vi "DeviceListCheck.vi"(0 "Device List":string[](array[string])=["9481_1", "9435_1", "9435_2", "9401_1", "9263_1", "9263_2"], 11 "Error In":errorcluster) -> (4 "Devices Present?":bool, 8 "Report Text":string, 15 "Error Out":errorcluster)   [LabVIEW 2023]
uses:
  <vilib>/nisyscfg/Find Hardware.vi
  <vilib>/nisyscfg/Close (System).vi
  <vilib>/nisyscfg/nisyscfg.lvlib
  <resource>/objmgr/nicontrollersysapi.rc
  <resource>/objmgr/pxisysapi.rc
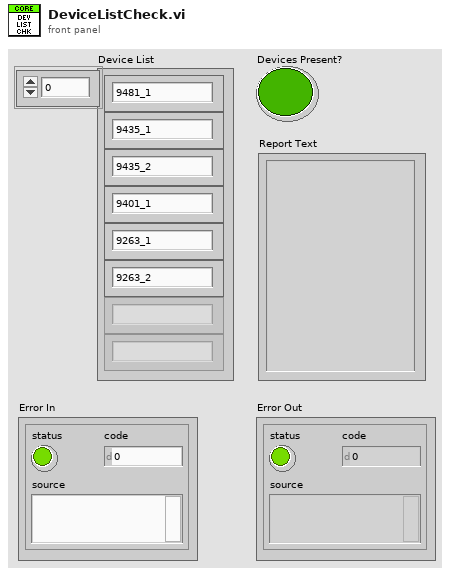
[diagram p1: front panel]
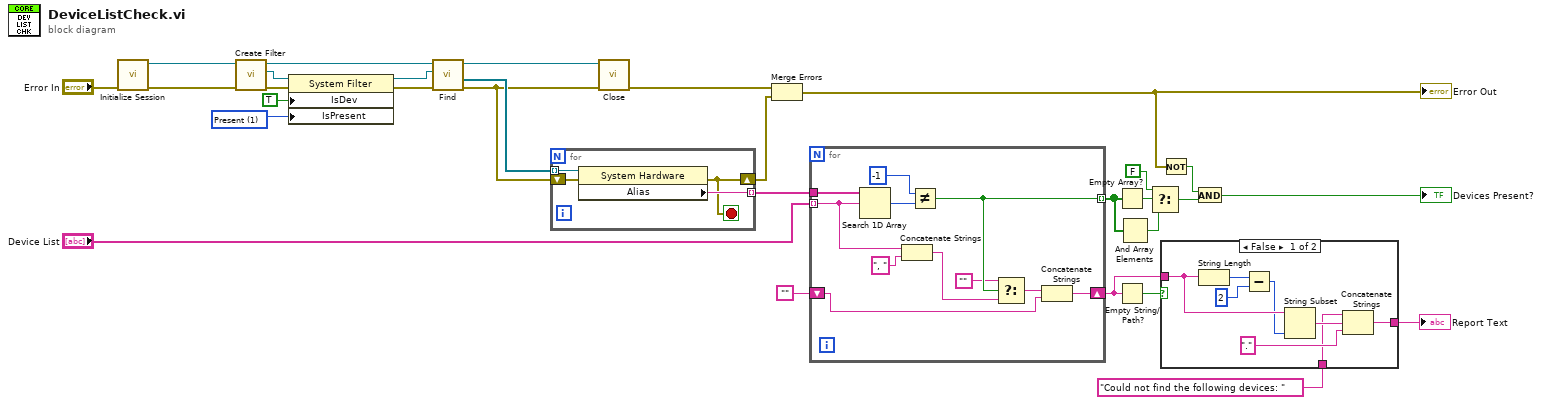
[diagram p0: block diagram]
diagram:
  w17 = 1 items=["Unknown"=-1, "Not Present"=0, "Present"=1] ("Devices & Chassis:Is Present")
  n1 = call <vilib>:"Initialize Session.vi"("error in (no error)"="Error In") -> ("error out"=w25:errorcluster, "Session out"=w24:refnum<k21>)  [unwired: 9 in]
  n2 = call <vilib>:"Create Filter.vi"("error in (no error)"=w25, "Session in"=w24) -> ("error out"=w28:errorcluster, "Filter out"=w27:refnum<k20>, "Session out"=w23:refnum<k21>)  [unwired: 7 in]
  n3 = property class="System Filter"(reference=w27, error in=w28, "IsDev"=TRUE ("Is Device"), "IsPresent"=w17) -> (reference out=w21:refnum<k20>, error out=w22:errorcluster)
  n4 = call-poly <vilib>:"Find.vi"("error in (no error)"=w22, "Filter in"=w21, "Session in"=w23) -> ("error out"=w16:errorcluster, "Resources out"=w29:refnum<k20>[], "Session out"=w30:refnum<k21>)  [unwired: 5 in, 1 out]
  n5 = for {
    tunnel: w29 -> [w34] mode=indexing
    tunnel: [w33] -> w20 mode=indexing
    shift-right: [w31] -> w14
    shift-left: w16 -> [w32]
    stop <- w31 stop-if-true
    n6 = property class="System Hardware"(reference=w34, error in=w32) -> (error out=w31:errorcluster, "Alias"=w33:string)  [unwired: 1 out]
  }
  n7 = call-poly <vilib>:"Close.vi"("error in (no error)"=w16, "Session in"=w30) -> ("error out"=w15:errorcluster)  [unwired: 9 in]
  n8 = Merge Errors(w15, w14) -> (w6:errorcluster)
  "Error Out" <- w6
  n9 = for {
    tunnel: w20 -> [w45]
    tunnel: "Device List" -> [w40] mode=indexing
    tunnel: [w42] -> w11 mode=indexing
    shift-right: [w35] -> w3
    shift-left: "" -> [w36]
    n10 = Search 1D Array(1D array=w45, element=w40) -> (index of element=w44:i32)  [unwired: 1 in]
    n11 = Concatenate Strings(w40, ", " ("string")) -> (w38:string)
    n12 = Not Equal?(x=-1, y=w44) -> (x != y?=w42:bool)
    n13 = Select(t="", s=w42, f=w38) -> (s? t:f=w37:string)
    n14 = Concatenate Strings(w37, w36) -> (w35:string)
  }
  n15 = Empty Array?(array=w11) -> (empty?=w13:bool)
  n16 = Empty String/Path?(string/path=w3) -> (empty?=w4:bool)
  n17 = And Array Elements(Boolean array=w11) -> (logical AND=w10:bool)
  n18 = Select(t=FALSE, s=w13, f=w10) -> (s? t:f=w9:bool)
  n19 = Not(x=w6) -> (.not. x?=w8:bool)
  n20 = case shown="False" w4 {
    tunnel: w3 -> [w51 w54]
    tunnel: "Could not find the following devices: " -> [w47 _]
    tunnel: [w46 w54] -> w1
    frame False {
      n21 = String Length(string=w51) -> (length=w53:i32)
      n22 = Subtract(x=w53, y=2) -> (x-y=w50:i32)
      n23 = String Subset(string=w51, length (rest)=w50) -> (substring=w49:string)  [unwired: 1 in]
      n24 = Concatenate Strings(w47, w49, "." ("substring (\"\")")) -> (w46:string)
    }
    frame True {
    }
  }
  "Report Text" <- w1
  n25 = And(x=w8, y=w9) -> (x .and. y?=→"Devices Present?":bool)
